vi "Popout Panel.vi"(8 "error in (no error)":errorcluster, 10 "Panel":refnum<class "Panel.lvclass">, 11 "PanelManager in":refnum<class "PanelManager.lvclass">) -> (0 "error out":errorcluster, 3 "PanelManager out":refnum<class "PanelManager.lvclass">)   [LabVIEW 2018, in "OOPanel.lvlib" / "PanelManager.lvclass"]
uses:
  PanelManager.lvclass
  Panel/Panel.lvclass
  Panel/State.ctl
  PanelManager.lvclass/PanelManager.ctl
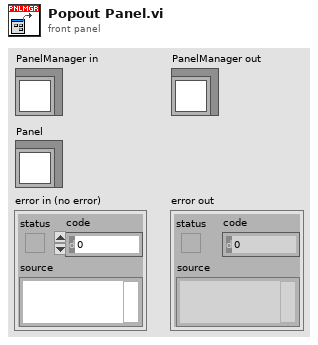
[diagram p1: front panel]
types:
  T1 = typedef "OOPanel.lvlib/Panel.lvclass/State.ctl" = enum16{"Idle", "Hidden", "Visible", "Subpanel"}
  T2 = typedef "OOPanel.lvlib/PanelManager.lvclass/Ref Data.ctl" = cluster{"Panels":T3, "Subpanel Map":T4}
  T3 = typedef "OOPanel.lvlib/PanelManager.lvclass/Panels.ctl" = cluster{"Names":string[], "Instances":refnum<class "Panel.lvclass">[]}
  T4 = typedef "OOPanel.lvlib/PanelManager.lvclass/SubPanel Map.ctl" = cluster{"SubPanels":refnum<vi>[], "Panels":refnum<class "Panel.lvclass">[]}
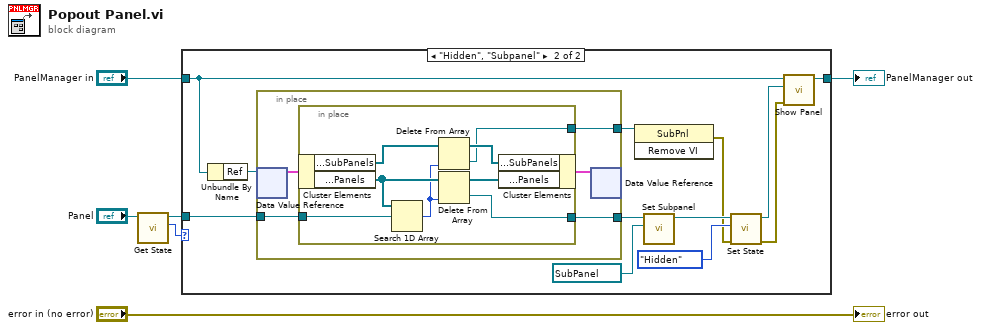
[diagram p0: block diagram]
diagram:
  n1 = call "Get State.vi"("Panel in"="Panel") -> ("State"=w1:T1, "Panel out"=w2:refnum<class "Panel.lvclass">)  [unwired: 8 in, 1 out]
  n2 = case shown="\"Hidden\", \"Subpanel\"" w1 {
    tunnel: w2 -> [_ w18]
    tunnel: "PanelManager in" -> [w7 w16]
    tunnel: [w7 w15] -> w4
    frame Default {
    }
    frame "Hidden", "Subpanel" {
      n3 = Unbundle By Name(w16) -> ("Ref"=w19:refnum<data-value>)
      n4 = in-place {
        in-place-border: w18 -> [w22]
        in-place-border: [w21] -> w14
        in-place-border: [w20] -> w17
        n5 = in-place-dvr #1(w19) -> (w24:T2)  [unwired: 1 out]
        n6 = in-place {
          in-place-border: w22 -> [w32]
          in-place-border: [w26] -> w21
          in-place-border: [w25] -> w20
          n7 = in-place-cluster #2(w24) -> ("Subpanel Map.SubPanels"=w30:refnum<vi>[], "Subpanel Map.Panels"=w31:refnum<class "Panel.lvclass">[])
          n8 = Search 1D Array(1D array=w31, element=w32) -> (index of element=w27:i32)  [unwired: 1 in]
          n9 = Delete From Array(array=w30, index=w27) -> (deleted portion=w25:refnum<vi>, array with subset deleted=w29:refnum<vi>[])  [unwired: 1 in]
          n10 = Delete From Array(array=w31, index=w27) -> (deleted portion=w26:refnum<class "Panel.lvclass">, array with subset deleted=w28:refnum<class "Panel.lvclass">[])  [unwired: 1 in]
          n11 = in-place-cluster #2("Subpanel Map.SubPanels"=w29, "Subpanel Map.Panels"=w28) -> (w23:T2)
        }
        n12 = in-place-dvr #1(w23) -> ()  [unwired: 2 out]
      }
      n13 = invoke class="SubPnl" method="Remove VI"(reference=w17) -> (error out=w10:errorcluster)  [unwired: 2 in, 2 out]
      n14 = call "Set Subpanel.vi"("Subpanel"=refnum<vi> refnum, "Panel in"=w14) -> ("Panel out"=w11:refnum<class "Panel.lvclass">)  [unwired: 8 in, 1 out]
      n15 = call "Set State.vi"("error in (no error)"=w10, "State"=State."Hidden", "Panel in"=w11) -> ("error out"=w8:errorcluster, "Panel out"=w9:refnum<class "Panel.lvclass">)  [unwired: 7 in]
      n16 = call-dynamic "Show Panel.vi"("error in (no error)"=w8, "Panel"=w9, "PanelManager in"=w16) -> ("PanelManager out"=w15:refnum<class "PanelManager.lvclass">)  [unwired: 7 in, 1 out]
    }
  }
  "PanelManager out" <- w4
  "error out" <- "error in (no error)"
